vi "TDD一致性检查.vi"(8 "TDD filePath":path, 9 "Spec String":string, 10 "SN":string, 11 "PN":string) -> (2 "报警颜色":string, 3 "判定":bool)   [LabVIEW 2011]
uses:
  <vilib>/Utility/config.llb/NI_LVConfig.lvlib
panel:
  in  "TDD":T1
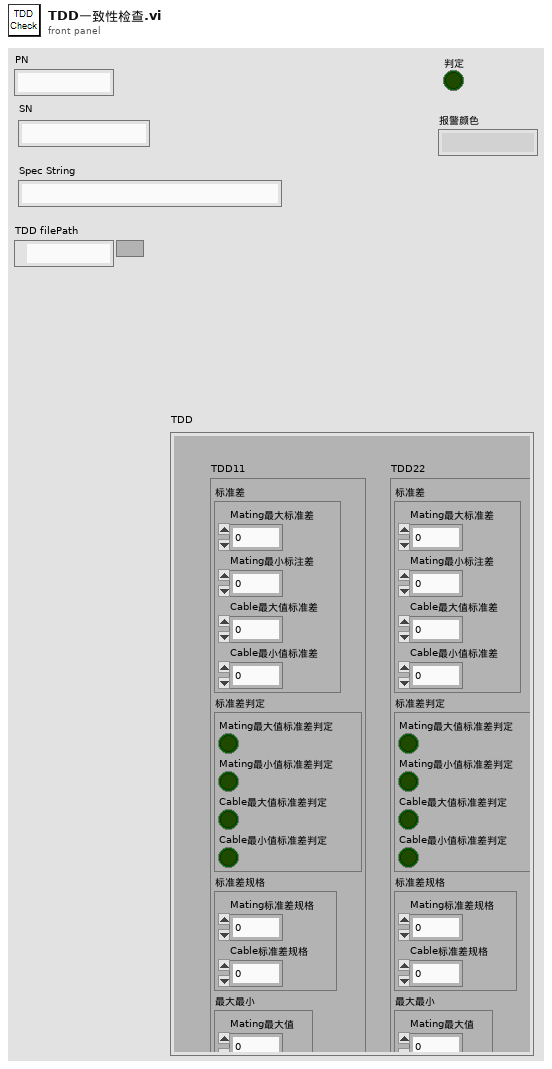
[diagram p1: front panel]
types:
  T1 = cluster{"TDD11":cluster{"标准差":cluster{"Mating最大标准差":dbl, "Mating最小标注差":dbl, "Cable最大值标准差":dbl, "Cable最小值标准差":dbl}, "标准差判定":cluster{"Mating最大值标准差判定":bool, "Mating最小值标准差判定":bool, "Cable最大值标准差判定":bool, "Cable最小值标准差判定":bool}, "标准差规格":cluster{"Mating标准差规格":dbl, "Cable标准差规格":dbl}, "最大最小":cluster{"Mating最大值":dbl, "Mating最小值":dbl, "Cable最大值":dbl, "Cable最小值":dbl}, "最大最小值判定":cluster{"Mating最小值判定":bool, "Mating最大值判定":bool, "Cable最大值判定":bool, "Cable最小值判定":bool}, "上下限规格":cluster{"MatingUpperValue":dbl, "MatingLowerValue":dbl, "CableUpperValue":dbl, "CableLowerValue":dbl}}, "TDD22":cluster{"标准差":cluster{"Mating最大标准差":dbl, "Mating最小标注差":dbl, "Cable最大值标准差":dbl, "Cable最小值标准差":dbl}, "标准差判定":cluster{"Mating最大值标准差判定":bool, "Mating最小值标准差判定":bool, "Cable最大值标准差判定":bool, "Cable最小值标准差判定":bool}, "标准差规格":cluster{"Mating标准差规格":dbl, "Cable标准差规格":dbl}, "最大最小":cluster{"Mating最大值":dbl, "Mating最小值":dbl, "Cable最大值":dbl, "Cable最小值":dbl}, "最大最小值判定":cluster{"Mating最小值判定":bool, "Mating最大值判定":bool, "Cable最大值判定":bool, "Cable最小值判定":bool}, "上下限规格":cluster{"MatingUpperValue":dbl, "MatingLowerValue":dbl, "CableUpperValue":dbl, "CableLowerValue":dbl}}}
  T2 = cluster{"标准差":cluster{"Mating最大标准差":dbl, "Mating最小标注差":dbl, "Cable最大值标准差":dbl, "Cable最小值标准差":dbl}, "标准差判定":cluster{"Mating最大值标准差判定":bool, "Mating最小值标准差判定":bool, "Cable最大值标准差判定":bool, "Cable最小值标准差判定":bool}, "标准差规格":cluster{"Mating标准差规格":dbl, "Cable标准差规格":dbl}, "最大最小":cluster{"Mating最大值":dbl, "Mating最小值":dbl, "Cable最大值":dbl, "Cable最小值":dbl}, "最大最小值判定":cluster{"Mating最小值判定":bool, "Mating最大值判定":bool, "Cable最大值判定":bool, "Cable最小值判定":bool}, "上下限规格":cluster{"MatingUpperValue":dbl, "MatingLowerValue":dbl, "CableUpperValue":dbl, "CableLowerValue":dbl}}
  T3 = cluster{"Mating最大值标准差判定":bool, "Mating最小值标准差判定":bool, "Cable最大值标准差判定":bool, "Cable最小值标准差判定":bool}
  T4 = cluster{"Mating最小值判定":bool, "Mating最大值判定":bool, "Cable最大值判定":bool, "Cable最小值判定":bool}
  T5 = typedef "NI_LVConfig.lvlib/Config Data RefNum.ctl" = refnum<k1>
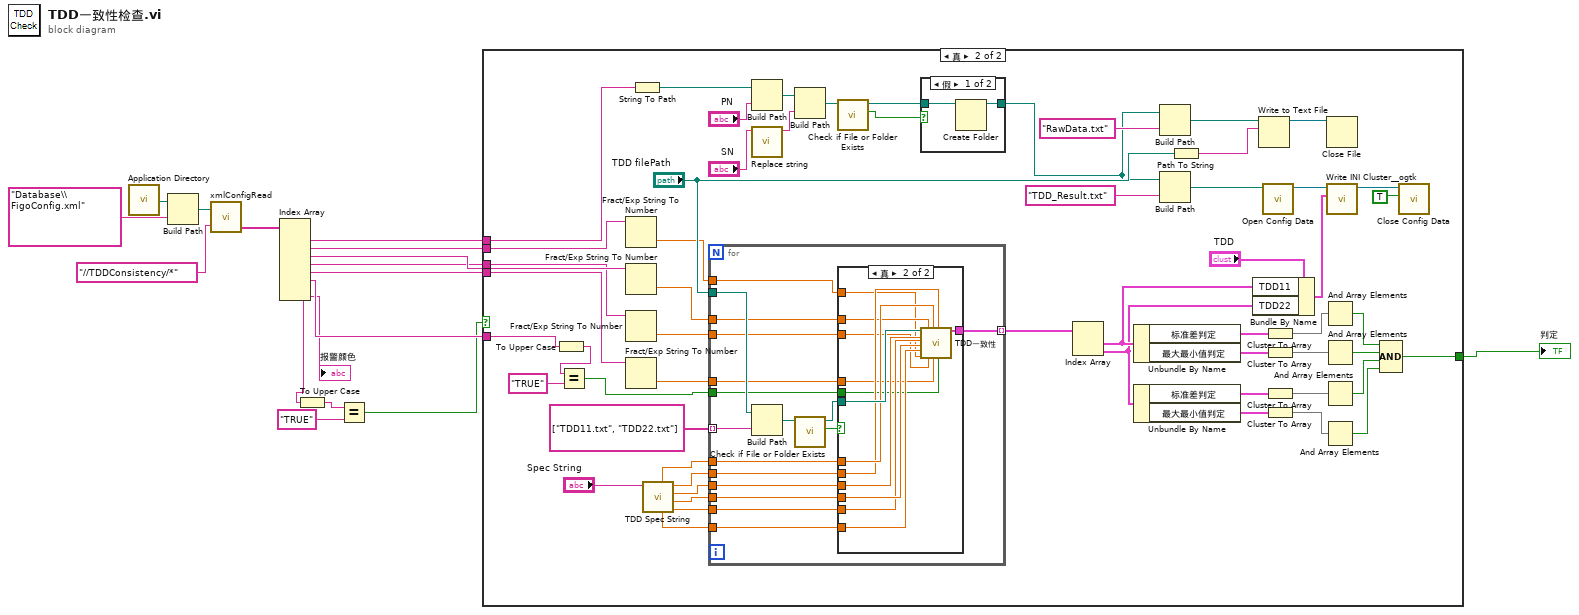
[diagram p0: block diagram]
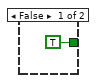
[diagram p2: hidden frame]
diagram:
  n1 = call <vilib>:"Application Directory.vi"() -> ("Application Directory"=w16:path)
  n2 = Build Path(base path=w16, name or relative path="Database\\FigoConfig.xml") -> (appended path=w14:path)
  n3 = call "xmlConfigRead.vi"("path to XML document"=w14, "XPath expression"="//TDDConsistency/*") -> ("OutParaArray"=w12:string[])  [unwired: 2 out]
  n4 = Index Array(array=w12) -> (element #1=w11:string, element #2=w10:string, element #3=w9:string, element #4=w8:string, element #5=w7:string, element #6=w6:string, element #7=w5:string, element #8=→"报警颜色":string)  [unwired: 8 in]
  n5 = To Upper Case(1:w5) -> (0:w4:string)
  n6 = Equal?(x=w4, y="TRUE") -> (x = y?=w2:bool)
  n7 = case shown="真" w2 {
    tunnel: [TRUE w33] -> w17
    tunnel: w11 -> [_ w32]
    tunnel: w10 -> [_ w30]
    tunnel: w9 -> [_ w28]
    tunnel: w8 -> [_ w26]
    tunnel: w7 -> [_ w24]
    tunnel: w6 -> [_ w22]
    frame False {
    }
    frame True {
      n8 = To Upper Case(1:w22) -> (0:w21:string)
      n9 = Equal?(x=w21, y="TRUE") -> (x = y?=w19:bool)
      n10 = Fract/Exp String To Number(string=w30) -> (number=w29:dbl)  [unwired: 3 in, 1 out]
      n11 = Fract/Exp String To Number(string=w28) -> (number=w27:dbl)  [unwired: 3 in, 1 out]
      n12 = Fract/Exp String To Number(string=w26) -> (number=w25:dbl)  [unwired: 3 in, 1 out]
      n13 = Fract/Exp String To Number(string=w24) -> (number=w23:dbl)  [unwired: 3 in, 1 out]
      n14 = String To Path(string=w32) -> (path=w31:path)
      n15 = call "TDD Spec String.vi"("Spec String"="Spec String") -> ("Mating LowerSpec"=w65:dbl, "Cable UpperSpec"=w66:dbl, "Mating UpperSpec"=w67:dbl, "CableArea"=w68:dbl, "Cable LowerSpec"=w64:dbl, "MatingArea"=w69:dbl)  [unwired: 5 in]
      n16 = for {
        tunnel: "TDD filePath" -> [w96]
        tunnel: string[] ["TDD11.txt", "TDD22.txt"] ("数组") -> [w95] mode=indexing
        tunnel: [w91] -> w72 mode=indexing
        tunnel: w69 -> [w90]
        tunnel: w68 -> [w89]
        tunnel: w67 -> [w88]
        tunnel: w66 -> [w87]
        tunnel: w65 -> [w86]
        tunnel: w64 -> [w85]
        tunnel: w27 -> [w84]
        tunnel: w29 -> [w83]
        tunnel: w25 -> [w82]
        tunnel: w23 -> [w81]
        tunnel: w19 -> [w80]
        n17 = Build Path(base path=w96, name or relative path=w95) -> (appended path=w94:path)
        n18 = call <vilib>:"Check if File or Folder Exists.vi"("path"=w94) -> ("file or folder exists?"=w93:bool, "dup path"=w92:path)  [unwired: 8 in, 1 out]
        n19 = case shown="真" w93 {
          tunnel: w92 -> [_ w109]
          tunnel: [_ w108] -> w91
          tunnel: w90 -> [_ w107]
          tunnel: w89 -> [_ w106]
          tunnel: w88 -> [_ w105]
          tunnel: w87 -> [_ w104]
          tunnel: w86 -> [_ w103]
          tunnel: w85 -> [_ w102]
          tunnel: w84 -> [_ w101]
          tunnel: w83 -> [_ w100]
          tunnel: w82 -> [_ w99]
          tunnel: w81 -> [_ w98]
          tunnel: w80 -> [_ w97]
          frame False {
          }
          frame True {
            n20 = call "TDD一致性.vi"("TDD filePath"=w109, "Mating Upper Spec"=w105, "Mating Lower Spec"=w103, "Cable Upper Spec"=w104, "Cable Lower Spec"=w102, "MatingPer"=w100, "CablePer"=w101, "Mating标准差规格"=w99, "Mating Area"=w107, "Cable标准差规格"=w98, "Cable Area"=w106, "Dialog"=w97) -> ("结果"=w108:T2)  [unwired: 6 in, 1 out]
          }
        }
      }
      n21 = Build Path(base path=w31, name or relative path="PN") -> (appended path=w48:path)
      n22 = call "Replace string.vi"("input string"="SN") -> ("output string"=w61:string)  [unwired: 10 in]
      n23 = Build Path(base path=w48, name or relative path=w61) -> (appended path=w53:path)
      n24 = call <vilib>:"Check if File or Folder Exists.vi"("path"=w53) -> ("file or folder exists?"=w52:bool, "dup path"=w51:path)  [unwired: 8 in, 1 out]
      n25 = case shown="假" w52 {
        tunnel: [w78 w79] -> w50
        tunnel: w51 -> [w77 w79]
        frame False {
          n26 = Create Folder(path (use dialog)=w77) -> (created path=w78:path)  [unwired: 2 in, 2 out]
        }
        frame True {
        }
      }
      n27 = Index Array(array=w72) -> (element #1=w47:T2, element #2=w46:T2)  [unwired: 2 in]
      n28 = Unbundle By Name(w47) -> ("标准差判定"=w45:T3, "最大最小值判定"=w44:T4)
      n29 = Unbundle By Name(w46) -> ("标准差判定"=w43:T3, "最大最小值判定"=w42:T4)
      n30 = Build Path(base path=w50, name or relative path="RawData.txt" ("名称或相对路径")) -> (appended path=w57:path)
      n31 = Build Path(base path=w50, name or relative path="TDD_Result.txt" ("名称或相对路径")) -> (appended path=w59:path)
      n32 = Path To String(path="TDD filePath") -> (string=w55:string)
      n33 = Bundle By Name(cluster="TDD", "TDD11"=w47, "TDD22"=w46) -> (w70:T1)
      n34 = Write to Text File(file (use dialog)=w57, text=w55) -> (refnum out=w54:refnum<file>)  [unwired: 2 in, 2 out]
      n35 = call <vilib>:"Open Config Data.vi"("configuration file path"=w59) -> ("refnum"=w75:T5)  [unwired: 8 in, 2 out]
      n36 = Cluster To Array(cluster=w45) -> (array=w41:bool[])
      n37 = Cluster To Array(cluster=w44) -> (array=w40:bool[])
      n38 = Cluster To Array(cluster=w43) -> (array=w39:bool[])
      n39 = Cluster To Array(cluster=w42) -> (array=w38:bool[])
      n40 = And Array Elements(Boolean array=w41) -> (logical AND=w37:bool)
      n41 = And Array Elements(Boolean array=w40) -> (logical AND=w36:bool)
      n42 = And Array Elements(Boolean array=w39) -> (logical AND=w35:bool)
      n43 = And Array Elements(Boolean array=w38) -> (logical AND=w34:bool)
      n44 = Close File(refnum=w54) -> ()  [unwired: 1 in, 2 out]
      n45 = call <userlib>:"Write INI Cluster__ogtk.vi"("INI Fomatted Cluster"=w70, "refnum"=w75) -> ("dup refnum"=w74:T5)  [unwired: 8 in, 1 out]
      n46 = Compound Arithmetic op=AND(w37, w36, w35, w34) -> (w33:bool)
      n47 = call <vilib>:"Close Config Data.vi"("write file if changed (T)"=TRUE, "refnum"=w74) -> ()  [unwired: 8 in, 2 out]
    }
  }
  "判定" <- w17
